vi "insert.vi"(8 "error in (no error)":errorcluster, 11 "DL090211ImageAssemblerScaffold in":refnum<class "ImageAssemblerRK110612Spiral.lvclass">) -> (0 "error out":errorcluster, 3 "DL090211ImageAssemblerScaffold out":refnum<class "ImageAssemblerRK110612Spiral.lvclass">)   [LabVIEW 2010, in "ImageAssemblerRK110612Spiral.lvclass"]
uses:
  ImageAssemblerRK110612Spiral.lvclass
  ImageAssemblerDL090211Scaffold/ImageAssemblerDL090211Scaffold/ImageAssemblerDL090211Scaffold.lvclass
  Analyser/GenericAnalyser/GenericAnalyser/GenericAnalyser.lvclass
  ImagingMode/GenericImagingMode/GenericImagingMode/trigger_enum.ctl
  ImagingMode/GenericImagingMode/GenericImagingMode/GenericImagingMode.lvclass
  DataCollection/GenericDataCollection/GenericDataCollection/GenericDataCollection.lvclass
  common/classes/Image/Image/Image.lvclass
  Display/GenericDisplay/GenericDisplay/GenericDisplay.lvclass
  common/classes/GenericComponent/GenericComponent/GenericComponent.lvclass
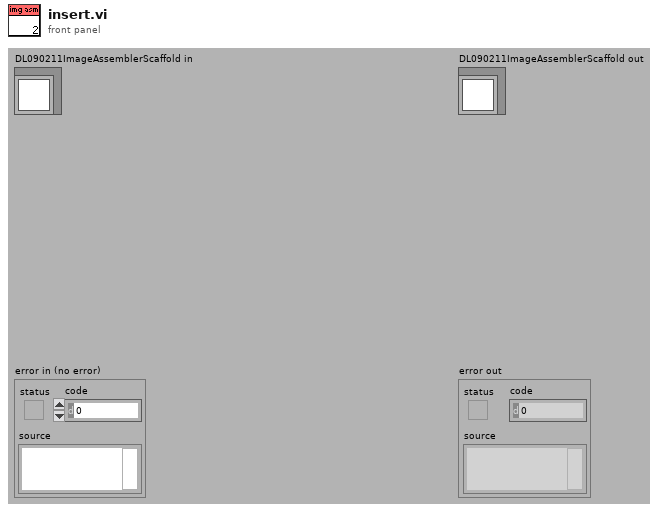
[diagram p1: front panel]
types:
  T1 = typedef "GenericImagingMode.lvclass/trigger_enum.ctl" = enum16{"NULL", "proceed"}
  T2 = typedef "IMAQ Image.ctl" = refnum<image>
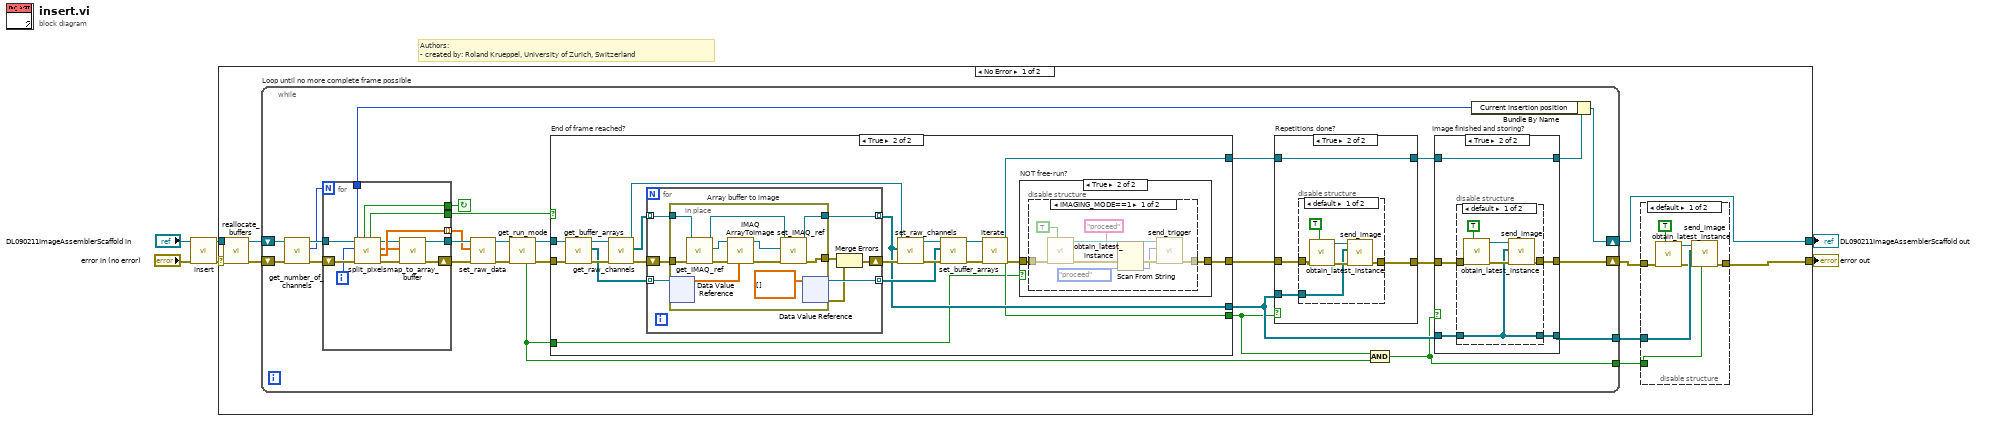
[diagram p0: block diagram]
diagram:
  # "Authors: \n- created by: Roland Krueppel, University of Zurich, Switzerland"
  n1 = call-parent "insert.vi"("error in (no error)"="error in (no error)", "ImageAssemblerDL090211Scaffold in"="DL090211ImageAssemblerScaffold in") -> ("error out"=w4:errorcluster, "ImageAssemblerDL090211Scaffold out"=w2:refnum<class "ImageAssemblerRK110612Spiral.lvclass">)  [unwired: 8 in]
  n2 = case shown="No Error" w4 {
    selector: w4 -> [w14 w146]
    tunnel: [w11 w146] -> w3
    tunnel: w2 -> [w15 w145]
    tunnel: [w7 w145] -> w1
    frame No Error {
      n3 = call-dynamic "reallocate_buffers.vi"("error in (no error)"=w14, "ImageAssemblerRK110612Spiral in"=w15) -> ("error out"=w13:errorcluster, "ImageAssemblerRK110612Spiral out"=w8:refnum<class "ImageAssemblerRK110612Spiral.lvclass">)  [unwired: 8 in]
      n4 = while "Loop until no more complete frame possible" {
        shift-right: [w32] -> w12
        shift-left: w13 -> [w43]
        tunnel: [w26] -> w10
        tunnel: [w25] -> w9
        shift-right: [w44] -> w7
        shift-left: w8 -> [w24]
        stop <- w48 continue-if-true
        n5 = call-dynamic "get_number_of_channels.vi"("error in (no error)"=w43, "GenericImageAssembler.lvclass in"=w24) -> ("error out"=w42:errorcluster, "number of channels"=w40:i32, "GenericImageAssembler.lvclass out"=w41:refnum<class "ImageAssemblerRK110612Spiral.lvclass">)  [unwired: 7 in]
        n6 = for {
          N: w40 -> [_]
          tunnel: w41 -> [w142]
          shift-right: [w136] -> w47
          shift-left: w42 -> [w144]
          tunnel: [w141] -> w45 mode=indexing
          tunnel: [w137] -> w50
          tunnel: [w135] -> w46
          tunnel: [w134] -> w49
          tunnel: [w133] -> w48
          i -> [w143]
          n7 = call-dynamic "split_pixels.vi"("error in (no error)"=w144, "Channel index"=w143, "ImageAssemblerRK110612Spiral in"=w142) -> ("error out"=w140:errorcluster, "For next frame"=w141:dbl[], "Pixel block"=w139:sgl[], "ImageAssemblerRK110612Spiral out"=w138:refnum<class "ImageAssemblerRK110612Spiral.lvclass">, "Next insertion position"=w137:i32, "End of frame reached?"=w134:bool, "Another frame possible?"=w133:bool)  [unwired: 2 in]
          n8 = call-dynamic "map_to_array_buffer.vi"("error in (no error)"=w140, "Pixel block"=w139, "ImageAssemblerRK110612Spiral in"=w138) -> ("error out"=w136:errorcluster, "ImageAssemblerRK110612Spiral out"=w135:refnum<class "ImageAssemblerRK110612Spiral.lvclass">)  [unwired: 7 in]
        }
        n9 = call-dynamic "set_raw_data.vi"("error in (no error)"=w47, "channels raw data block"=w45, "GenericImageAssembler.lvclass in"=w46) -> ("error out"=w34:errorcluster, "GenericImageAssembler.lvclass out"=w37:refnum<class "ImageAssemblerRK110612Spiral.lvclass">)  [unwired: 7 in]
        n10 = call "get_run_mode.vi"("error in (no error)"=w34, "GenericPlugin in"=w37) -> ("error out"=w35:errorcluster, "GenericPlugin out"=w36:refnum<class "ImageAssemblerRK110612Spiral.lvclass">, "is NOT free run?"=w27:bool)  [unwired: 5 in, 2 out]
        n11 = case "End of frame reached?" shown="True" w49 {
          tunnel: w35 -> [w80 w88]
          tunnel: [w80 w81] -> w38
          tunnel: w36 -> [w79 w89]
          tunnel: [_ w83] -> w28
          tunnel: [w79 w86] -> w39
          tunnel: [_ w90] -> w29
          tunnel: w27 -> [_ w82]
          frame False {
          }
          frame True {
            n12 = call-dynamic "get_buffer_arrays.vi"("error in (no error)"=w88, "ImageAssemblerRK110612Spiral in"=w89) -> ("error out"=w97:errorcluster, "Buffer arrays"=w96:refnum<data-value>[], "ImageAssemblerRK110612Spiral out"=w98:refnum<class "ImageAssemblerRK110612Spiral.lvclass">)  [unwired: 7 in]
            n13 = call-dynamic "get_raw_channels.vi"("error in (no error)"=w97, "DL090211ImageAssemblerScaffold.lvclass in"=w98) -> ("error out"=w100:errorcluster, "raw channels"=w99:refnum<class "Image.lvclass">[], "DL090211ImageAssemblerScaffold.lvclass out"=w93:refnum<class "ImageAssemblerRK110612Spiral.lvclass">)  [unwired: 7 in]
            n14 = for {
              tunnel: [w121] -> w90 mode=indexing
              tunnel: w96 -> [w120] mode=indexing
              tunnel: [w119] -> w91 mode=indexing
              shift-right: [w116] -> w95
              shift-left: w100 -> [w118]
              tunnel: w99 -> [w117] mode=indexing
              n15 = in-place "Array buffer to image" {
                in-place-border: w118 -> [w132]
                in-place-border: w117 -> [w130]
                in-place-border: [w127] -> w115
                in-place-border: [w124] -> w121
                n16 = in-place-dvr #1(w120) -> (w123:sgl[][])  [unwired: 1 out]
                n17 = call-dynamic "get_IMAQ_ref.vi"("error in (no error)"=w132, "Image.lvclass in"=w130) -> ("error out"=w131:errorcluster, "Image"=w129:T2, "Image.lvclass out"=w126:refnum<class "Image.lvclass">)  [unwired: 5 in, 2 out]
                n18 = call "IMAQ ArrayToImage"("Image Pixels (Float)"=w123, "error in (no error)"=w131, "Image"=w129) -> ("error out"=w128:errorcluster, "Image Out"=w125:T2)  [unwired: 7 in]
                n19 = call-dynamic "set_IMAQ_ref.vi"("error in (no error)"=w128, "Image"=w125, "Image.lvclass in"=w126) -> ("error out"=w127:errorcluster, "Image.lvclass out"=w124:refnum<class "Image.lvclass">)  [unwired: 7 in]
                n20 = in-place-dvr #1(sgl[][] [] ("data value")) -> (w119:refnum<data-value>, w114:errorcluster)
              }
              n21 = Merge Errors(w115, w114) -> (w116:errorcluster)
            }
            n22 = call "set_raw_channels.vi"("error in (no error)"=w95, "raw channels"=w90, "DL090211ImageAssemblerScaffold.lvclass in"=w93) -> ("error out"=w94:errorcluster, "DL090211ImageAssemblerScaffold.lvclass out"=w92:refnum<class "ImageAssemblerRK110612Spiral.lvclass">)  [unwired: 7 in]
            n23 = call-dynamic "set_buffer_arrays.vi"("error in (no error)"=w94, "Buffer arrays"=w91, "ImageAssemblerRK110612Spiral in"=w92) -> ("error out"=w85:errorcluster, "ImageAssemblerRK110612Spiral out"=w87:refnum<class "ImageAssemblerRK110612Spiral.lvclass">)  [unwired: 7 in]
            n24 = call-dynamic "iterate.vi"("error in (no error)"=w85, "DL090211ImageAssemblerScaffold in"=w87) -> ("error out"=w84:errorcluster, "finished?"=w83:bool, "DL090211ImageAssemblerScaffold out"=w86:refnum<class "ImageAssemblerRK110612Spiral.lvclass">)  [unwired: 7 in]
            n25 = case "NOT free-run?" shown="True" w82 {
              tunnel: w84 -> [w101 w103]
              tunnel: [w101 w102] -> w81
              frame False {
              }
              frame True {
                n26 = disable-structure shown="IMAGING_MODE==1" {
                  disable-tunnel: w103 -> [w111 w113]
                  disable-tunnel: [w112 w113] -> w102
                  frame condition #0 {
                    n27 = call "obtain_latest_instance.vi"("quick, but maybe outdated?"=TRUE, "error in (no error)"=w111) -> ("error out"=w108:errorcluster, "GenericScanMode out"=w110:refnum<class "GenericImagingMode.lvclass">)  [unwired: 8 in]
                    n28 = Scan From String(input string="proceed", error in=w108, default 1=trigger_enum."proceed" ("message")) -> (error out=w107:errorcluster, output 1=w106:T1)  [unwired: 2 in, 2 out]
                    n29 = call-dynamic "send_trigger.vi"("error in (no error)"=w107, "message"=w106, "GenericScanMode in"=w110) -> ("error out"=w112:errorcluster)  [unwired: 8 out]
                  }
                  frame condition #1 (active) {
                  }
                }
              }
            }
          }
        }
        n30 = case "Repetitions done?" shown="True" w28 {
          tunnel: w38 -> [w66 w71]
          tunnel: w39 -> [w67 w68]
          tunnel: [w66 w70] -> w33
          tunnel: [w67 w68] -> w31
          tunnel: w29 -> [_ w69]
          frame False {
          }
          frame True {
            n31 = disable-structure shown="default" {
              disable-tunnel: w71 -> [w74 w78]
              disable-tunnel: [w73 w78] -> w70
              disable-tunnel: w69 -> [w72 _]
              frame condition #0 (active) {
                n32 = call "obtain_latest_instance.vi"("quick, but maybe outdated?"=TRUE, "error in (no error)"=w74) -> ("error out"=w76:errorcluster, "GeneralAnalyser out"=w75:refnum<class "GenericAnalyser.lvclass">)  [unwired: 8 out]
                n33 = call-dynamic "send_image.vi"("error in (no error)"=w76, "image (channels)"=w72, "GenericToplevelComponent in"=w75) -> ("error out"=w73:errorcluster)  [unwired: 2 in, 6 out]
              }
              frame condition #1 {
              }
            }
          }
        }
        n34 = And(x=w28, y=w27) -> (x .and. y?=w26:bool)
        n35 = case "Image finished and storing?" shown="True" w26 {
          tunnel: w33 -> [w52 w58]
          tunnel: [w52 w57] -> w32
          tunnel: w29 -> [w51 w56]
          tunnel: w31 -> [w53 w55]
          tunnel: [w53 w55] -> w30
          tunnel: [w51 w54] -> w25
          frame False {
          }
          frame True {
            n36 = disable-structure shown="default" {
              disable-tunnel: w58 -> [w63 _]
              disable-tunnel: [w64 _] -> w57
              disable-tunnel: w56 -> [w60 w65]
              disable-tunnel: [w60 w65] -> w54
              frame condition #0 (active) {
                n37 = call "obtain_latest_instance.vi"("quick, but maybe outdated?"=TRUE, "error in (no error)"=w63) -> ("error out"=w62:errorcluster, "GenericDataCollection out"=w61:refnum<class "GenericDataCollection.lvclass">)  [unwired: 8 out]
                n38 = call-dynamic "send_image.vi"("error in (no error)"=w62, "image (channels)"=w60, "GenericToplevelComponent in"=w61) -> ("error out"=w64:errorcluster)  [unwired: 2 in, 6 out]
              }
              frame condition #1 {
              }
            }
          }
        }
        n39 = Bundle By Name(cluster=w30, "Current insertion position"=w50) -> (w44:refnum<class "ImageAssemblerRK110612Spiral.lvclass">)
      }
      n40 = disable-structure shown="default" {
        disable-tunnel: w9 -> [w22 _]
        disable-tunnel: [w21 w23] -> w11
        disable-tunnel: w12 -> [w19 w23]
        disable-tunnel: w10 -> [w16 _]
        frame condition #0 (active) {
          n41 = call "obtain_latest_instance.vi"("quick, but maybe outdated?"=TRUE, "error in (no error)"=w19) -> ("error out"=w18:errorcluster, "GenericDisplay out"=w20:refnum<class "GenericDisplay.lvclass">)  [unwired: 8 out]
          n42 = call-dynamic "send_image.vi"(6:w16, "error in (no error)"=w18, "image (channels)"=w22, "GenericToplevelComponent in"=w20) -> ("error out"=w21:errorcluster)  [unwired: 2 in, 5 out]
        }
        frame condition #1 {
        }
      }
    }
    frame Error {
    }
  }
  "error out" <- w3
  "DL090211ImageAssemblerScaffold out" <- w1
